vi "Intan_VerifySerialLink.vi"(8 "error in":errorcluster, 11 "VISA resource name":refnum<visa-resource-name>="COM1") -> (0 "error out":errorcluster, 2 "Text response":string, 3 "VISA resource name out":refnum<visa-resource-name>)   [LabVIEW 2017]
panel:
  in  "bytes to read":u32=1000
  out "return count":u32
  in  "Teensy event char":string="v"
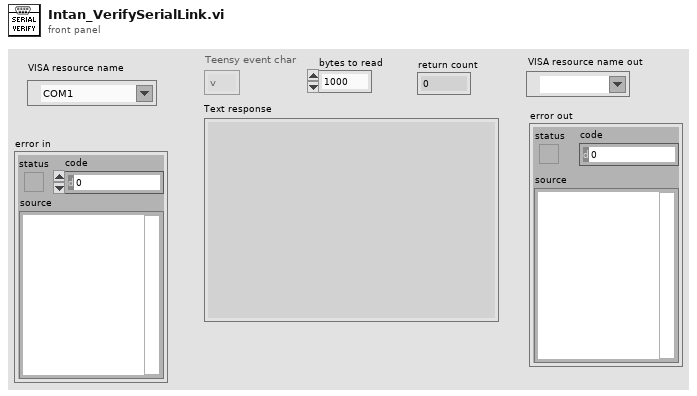
[diagram p1: front panel]
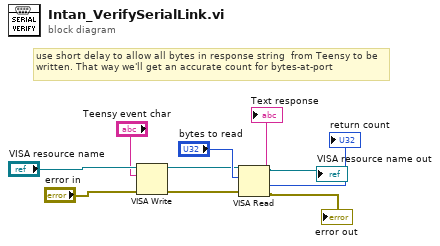
[diagram p0: block diagram]
diagram:
  # "use short delay to allow all bytes in response string  from Teensy to be written. That way we'll get an accurate count for bytes-at-port"
  n1 = VISA Write(VISA resource name="VISA resource name", write buffer="Teensy event char", error in (no error)="error in") -> (VISA resource name out=w3:refnum<visa-resource-name>, error out=w2:errorcluster)  [unwired: 1 out]
  n2 = VISA Read(VISA resource name=w3, byte count="bytes to read", error in (no error)=w2) -> (VISA resource name out=→"VISA resource name out":refnum<visa-resource-name>, read buffer=→"Text response":string, return count=→"return count":u32, error out=→"error out":errorcluster)
